vi "Confirm GU Arrange Scheme.vi"(8 "error in":errorcluster, 9 "Error Cell":T3(array[cluster]), 10 "Curr Cal Cfg In":T1, 11 "GU Arrange List":refnum<vi>) -> (0 "error out":errorcluster, 2 "Curr Cal Cfg Out":T1, 3 "GU Arrange List  Ref Out":refnum<vi>, 5 "Next Event":string)   [LabVIEW 2020, in "GUCalibration2.lvlib"]
uses:
  GUCalibration2.lvlib
  Controls/Config Data Type.ctl
  Controls/GU Arrange Check Rule.ctl
  Controls/User Facing Msg Enum.ctl
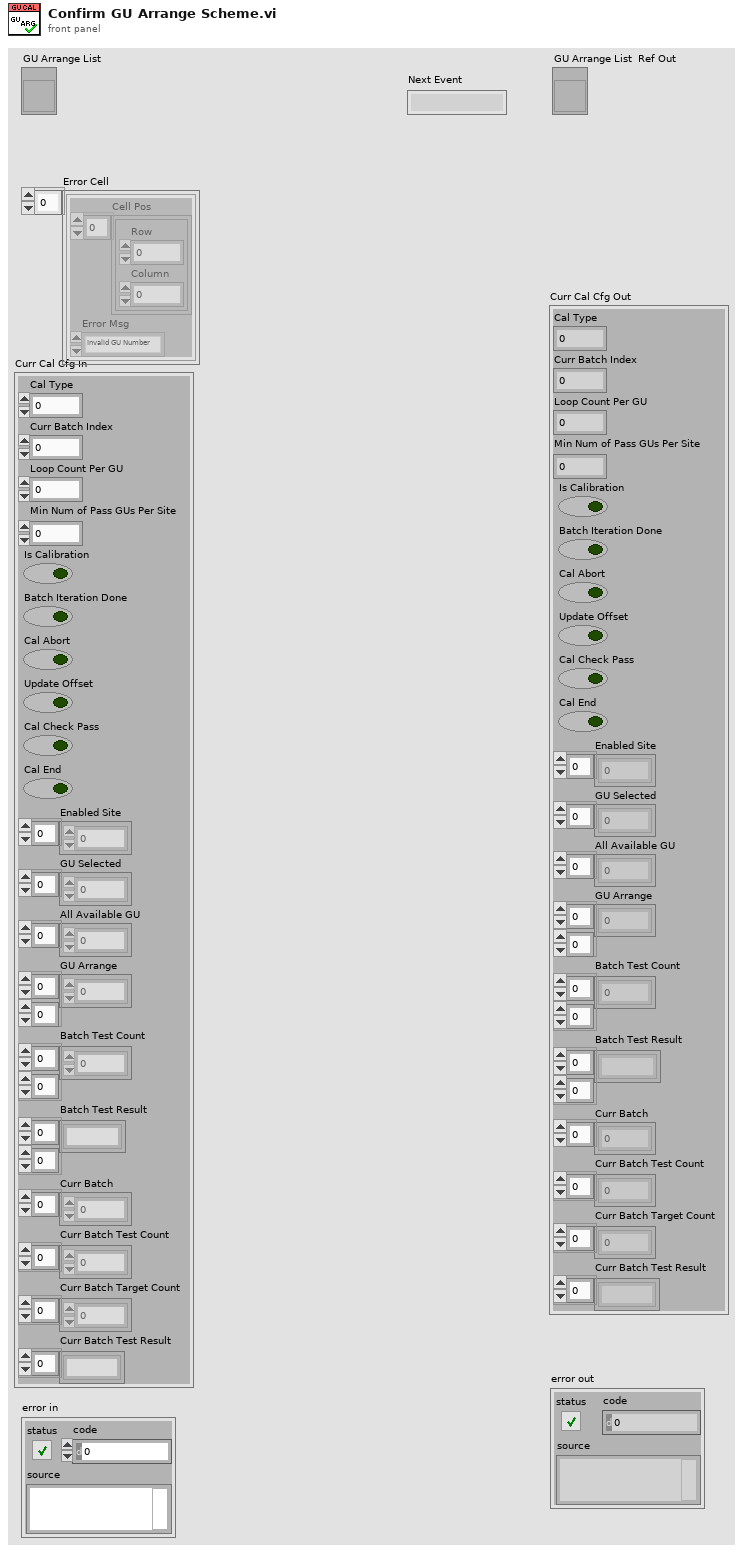
[diagram p1: front panel]
types:
  T1 = typedef "GUCalibration2.lvlib/Config Data Type.ctl" = cluster{"Cal Type":i32, "Curr Batch Index":i32, "Loop Count Per GU":i32, "Min Num of Pass GUs Per Site":i32, "Is Calibration":bool, "Batch Iteration Done":bool, "Cal Abort":bool, "Update Offset":bool, "Cal Check Pass":bool, "Cal End":bool, "Enabled Site":i32[], "GU Selected":i32[], "All Available GU":i32[], "GU Arrange":i32[][], "Batch Test Count":i32[][], "Batch Test Result":string[][], "Curr Batch":i32[], "Curr Batch Test Count":i32[], "Curr Batch Target Count":i32[], "Curr Batch Test Result":string[]}
  T2 = typedef "GUCalibration2.lvlib/GU Arrange Check Rule.ctl" = enum16{"Invalid GU Number", "GU Number Conflict"}
  T3 = cluster{"Cell Pos":cluster{"Row":i32, "Column":i32}[], "Error Msg":T2}[]
  T4 = typedef "GUCalibration2.lvlib/User Facing Msg Enum.ctl" = enum16{"Invalid GU Number", "Select More GU", "Exceptional Lot End", "Not All Sites Test", "GU Arrange Error", "Put GU In Sites", "No Cal Site Offset Msg"}
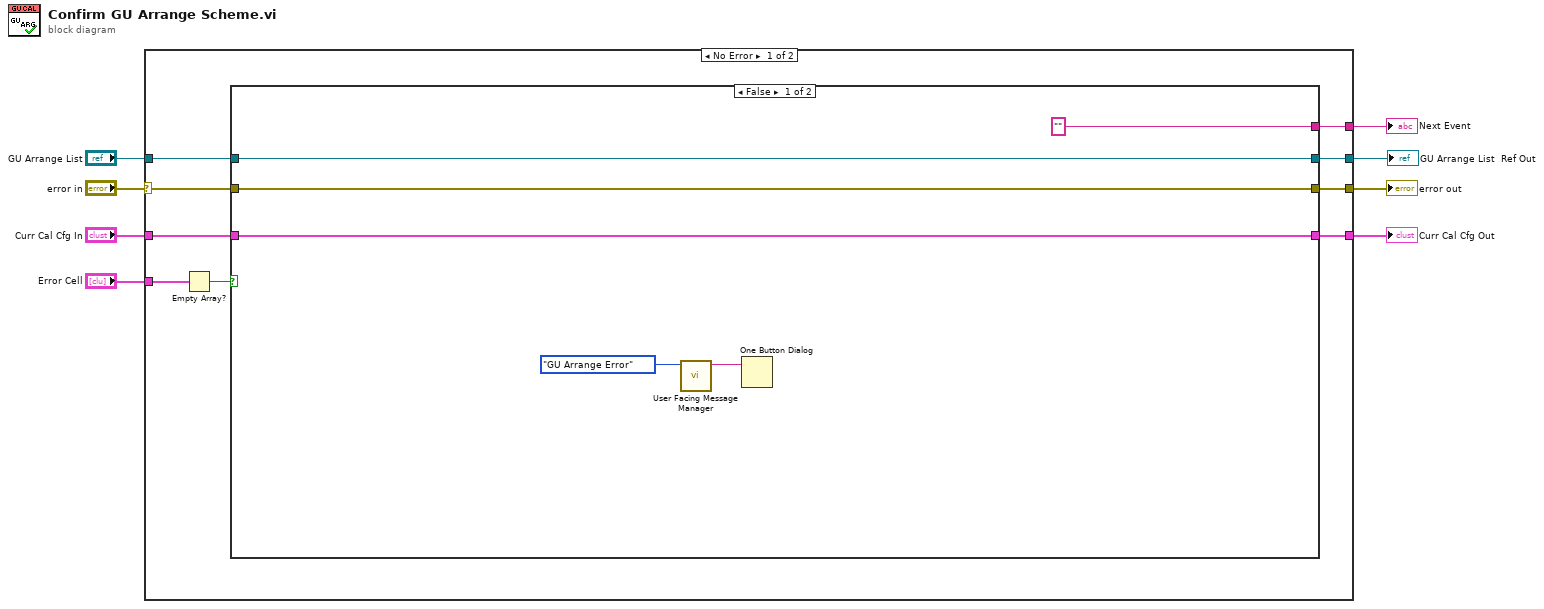
[diagram p0: block diagram]
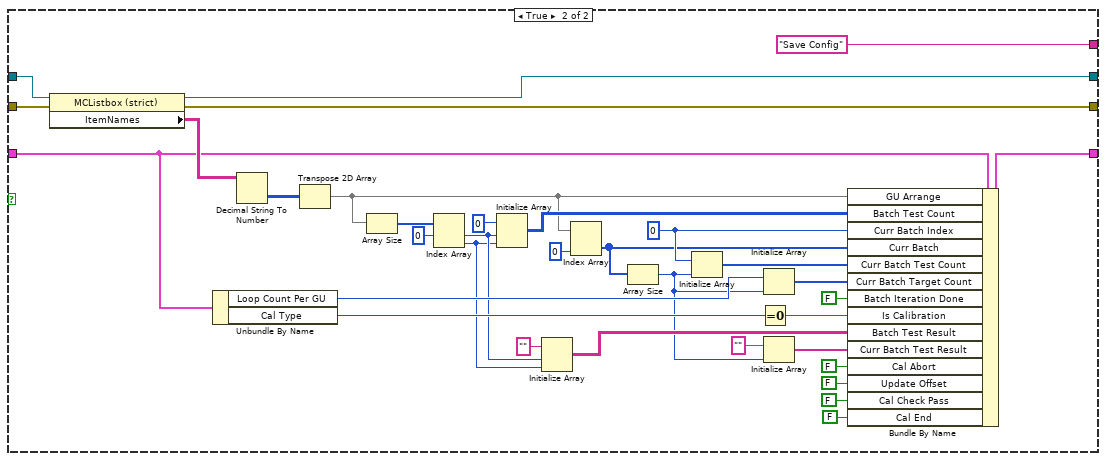
[diagram p2: hidden frame]
diagram:
  n1 = case shown="No Error" "error in" {
    selector: "error in" -> [w14 w59]
    tunnel: "GU Arrange List" -> [w17 w58]
    tunnel: "Curr Cal Cfg In" -> [w15 w60]
    tunnel: [w16 w59] -> w7
    tunnel: [w12 w60] -> w5
    tunnel: [w13 w58] -> w4
    tunnel: "Error Cell" -> [w11 _]
    tunnel: [w9 _] -> w1
    frame No Error {
      n2 = Empty Array?(array=w11) -> (empty?=w10:bool)
      n3 = case shown="False" w10 {
        tunnel: w17 -> [w21 w57]
        tunnel: [w23 w56] -> w16
        tunnel: w15 -> [w22 w41]
        tunnel: w14 -> [w23 w55]
        tunnel: [w21 w54] -> w13
        tunnel: [w22 w52] -> w12
        tunnel: ["" ("message") "Save Config" ("message")] -> w9
        frame False {
          n4 = call "User Facing Message Manager.vi"("User Facing Msg"=User_Facing_Msg_Enum."GU Arrange Error") -> ("User Facing Msg Out"=w18:string)  [unwired: 8 in, 2 out]
          n5 = One Button Dialog(message=w18) -> ()  [unwired: 1 in, 1 out]
        }
        frame True {
          w45 = 0 ("Curr GU Index")
          n6 = property class="MCListbox (strict)"(reference=w57, error in=w55) -> (reference out=w54:refnum<vi>, error out=w56:errorcluster, "ItemNames"=w53:string[][])
          n7 = Unbundle By Name(w41) -> ("Loop Count Per GU"=w40:i32, "Cal Type"=w36:i32)
          n8 = Decimal String To Number(string=w53) -> (number=w48:i32[][])  [unwired: 2 in, 1 out]
          n9 = Transpose 2D Array(2D array=w48) -> (transposed array=w42:i32[][])
          n10 = Array Size(array=w42) -> (size(s)=w51:i32[])
          n11 = Index Array(array=w51, index #1=0 ("index")) -> (element #1=w34:i32, element #2=w33:i32)  [unwired: 1 in]
          n12 = Initialize Array(0 ("index"), w34, w33) -> (w47:i32[][])
          n13 = Initialize Array("", w34, w33) -> (w31:string[][])
          n14 = Index Array(array=w42, index (col)=0 ("disabled index (col)")) -> (element=w44:i32[])  [unwired: 1 in]
          n15 = Array Size(array=w44) -> (size(s)=w30:i32)
          n16 = Initialize Array(w45, w30) -> (w43:i32[])
          n17 = Equal To 0?(x=w36) -> (x = 0?=w35:bool)
          n18 = Initialize Array(w40, w30) -> (w39:i32[])
          n19 = Initialize Array("", w30) -> (w28:string[])
          n20 = Bundle By Name(cluster=w41, "GU Arrange"=w42, "Batch Test Count"=w47, "Curr Batch Index"=w45, "Curr Batch"=w44, "Curr Batch Test Count"=w43, "Curr Batch Target Count"=w39, "Batch Iteration Done"=FALSE ("Calibration End"), "Is Calibration"=w35, "Batch Test Result"=w31, "Curr Batch Test Result"=w28, "Cal Abort"=FALSE, "Update Offset"=FALSE, "Cal Check Pass"=FALSE, "Cal End"=FALSE) -> (w52:T1)
        }
      }
    }
    frame Error {
    }
  }
  "error out" <- w7
  "Curr Cal Cfg Out" <- w5
  "GU Arrange List  Ref Out" <- w4
  "Next Event" <- w1
